vi "DataNameFormats.vi"(8 "ErrorIn(No Error)":errorcluster caption="entrée d'erreur (pas d'erreur)", 10 "InstrumentName":string, 11 "DataNameArr":string[](array[string])) -> (0 "Err Out":errorcluster caption="sortie d'erreur", 3 "DataNameArrOut":string[](array[string]))   [LabVIEW 2019]
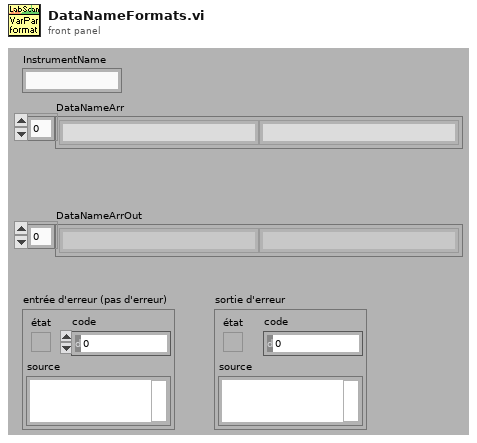
[diagram p1: front panel]
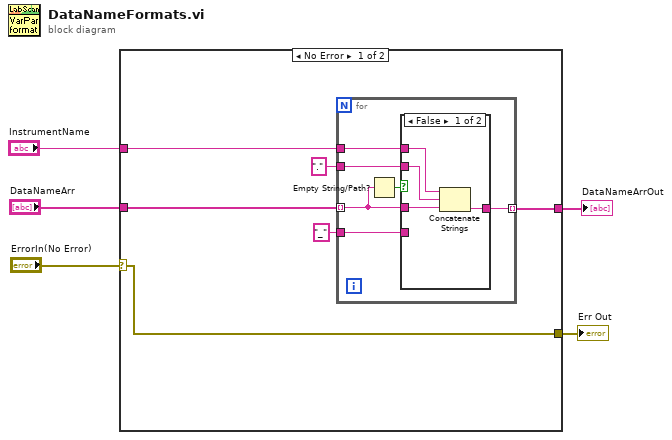
[diagram p0: block diagram]
diagram:
  n1 = case shown="No Error" "ErrorIn(No Error)" {
    selector: "ErrorIn(No Error)" -> [w8 w23]
    tunnel: [w8 w23] -> w4
    tunnel: "InstrumentName" -> [w11 _]
    tunnel: "DataNameArr" -> [w10 _]
    tunnel: [w9 _] -> w1
    frame No Error {
      n2 = for {
        tunnel: w10 -> [w12] mode=indexing
        tunnel: "." ("chaîne") -> [w17]
        tunnel: [w16] -> w9 mode=indexing
        tunnel: w11 -> [w15]
        tunnel: "_" ("chaîne") -> [w14]
        n3 = Empty String/Path?(string/path=w12) -> (empty?=w13:bool)
        n4 = case shown="False" w13 {
          tunnel: w12 -> [w21 w22]
          tunnel: w17 -> [w20 _]
          tunnel: [w19 w22] -> w16
          tunnel: w15 -> [w18 _]
          tunnel: w14 -> [_ _]
          frame False {
            n5 = Concatenate Strings(w18, w20, w21) -> (w19:string)
          }
          frame True {
          }
        }
      }
    }
    frame Error {
    }
  }
  "Err Out" <- w4
  "DataNameArrOut" <- w1
